vi "EncodeInt8.vi"(1 "Data In":i8[](array[numeric])) -> (0 "Data Out":u8[](array[numeric]))   [LabVIEW 2014, in "navX-MXP IMU.lvlib"]
uses:
  navX-MXP IMU.lvlib
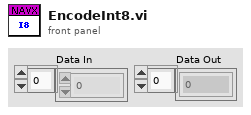
[diagram p1: front panel]
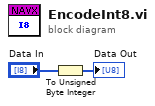
[diagram p0: block diagram]
diagram:
  n1 = To Unsigned Byte Integer(number="Data In") -> (unsigned 8bit integer=→"Data Out":u8[])
